vi "Get base-path.vi"(6 "Strip lead \"/\" (F)":bool, 8 "error in (no error)":errorcluster, 11 "URI-Component.Path in":refnum<class "URI-Component.Path.lvclass">) -> (0 "error out":errorcluster, 2 "base-path":string, 3 "URI-Component.Path out":refnum<class "URI-Component.Path.lvclass">)   [LabVIEW 2013, in "openURI.lvlib" / "URI-Component.Path.lvclass"]
uses:
  URI-Component.Path.lvclass
  URI-Component.Path.lvclass/URI-Component.Path.ctl
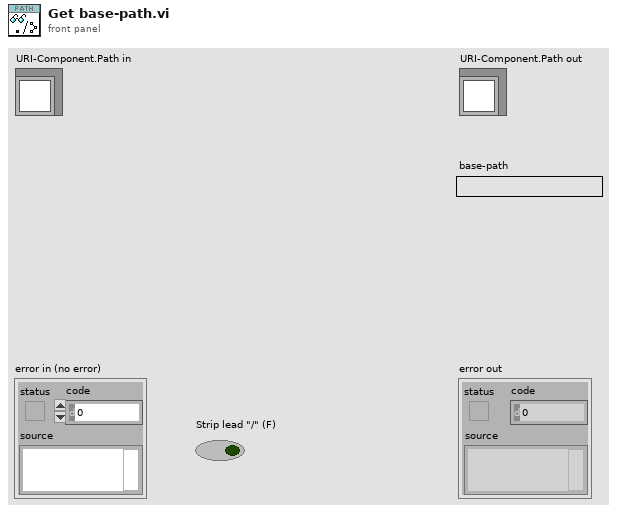
[diagram p1: front panel]
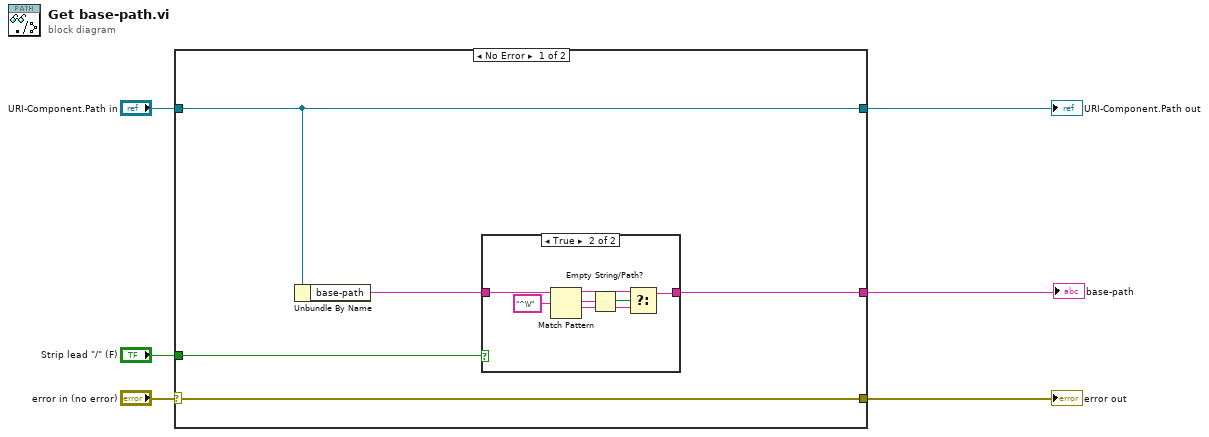
[diagram p0: block diagram]
diagram:
  n1 = case shown="No Error" "error in (no error)" {
    selector: "error in (no error)" -> [w11 w21]
    tunnel: [w11 w21] -> w5
    tunnel: [w8 w20] -> w3
    tunnel: "URI-Component.Path in" -> [w8 w20]
    tunnel: [w7 _] -> w2
    tunnel: "Strip lead \"/\" (F)" -> [w10 _]
    frame No Error {
      n2 = Unbundle By Name(w8) -> ("base-path"=w9:string)
      n3 = case shown="True" w10 {
        tunnel: [w12 w13] -> w7
        tunnel: w9 -> [w12 w19]
        frame False {
        }
        frame True {
          n4 = Match Pattern(string=w19, regular expression="^\\/") -> (before substring=w15:string, match substring=w17:string, after substring=w14:string)  [unwired: 1 in, 1 out]
          n5 = Empty String/Path?(string/path=w17) -> (empty?=w16:bool)
          n6 = Select(t=w15, s=w16, f=w14) -> (s? t:f=w13:string)
        }
      }
    }
    frame Error {
    }
  }
  "error out" <- w5
  "URI-Component.Path out" <- w3
  "base-path" <- w2
